vi "Voltage Cycle.vi"() -> ()   [LabVIEW 2015]
uses:
  <instrlib>/Agilent E363X Series/Agilent E363X Series.lvlib
panel:
  in  "Delay Control":dbl format="%#_g seconds"
  in  "Ending Voltage":dbl format="%#_g V"
  in  "Voltage Step":dbl format="%#_g V"
  out "# Trials":dbl
  in  "Dosimeter Id":string
  in  "Starting Voltage":dbl format="%#_g V"
  out "?":bool
  in  "Current Limit (1.0 A)":dbl=1.0 format="%.3g"
  out "Actual Current Level (A)":dbl format="%.3g"
  in  "Channel (1: Channel 1)":i32(ring)=1 items=["Channel 1"=1, "Channel 2"=2, "Channel 3"=3]
  out "Actual Voltage Level (V)":dbl format="%.3g"
  in  "VISA resource name":refnum<visa-resource-name>
  in  "?":bool
  in  "# Measurements":dbl format="%#_g "
  in  "Time inbetween Trials":dbl format="%#_g seconds"
  in  "Time inbetween Measurements":dbl format="%#_g seconds"
  out "Output":string="Start Ipad"
  out "Voltage":dbl(knob) scale=0.0..6.0
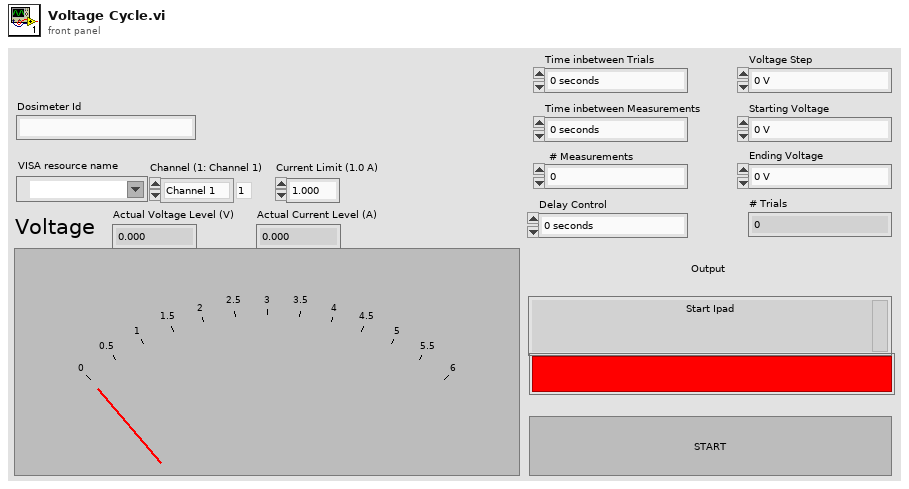
[diagram p1: front panel]
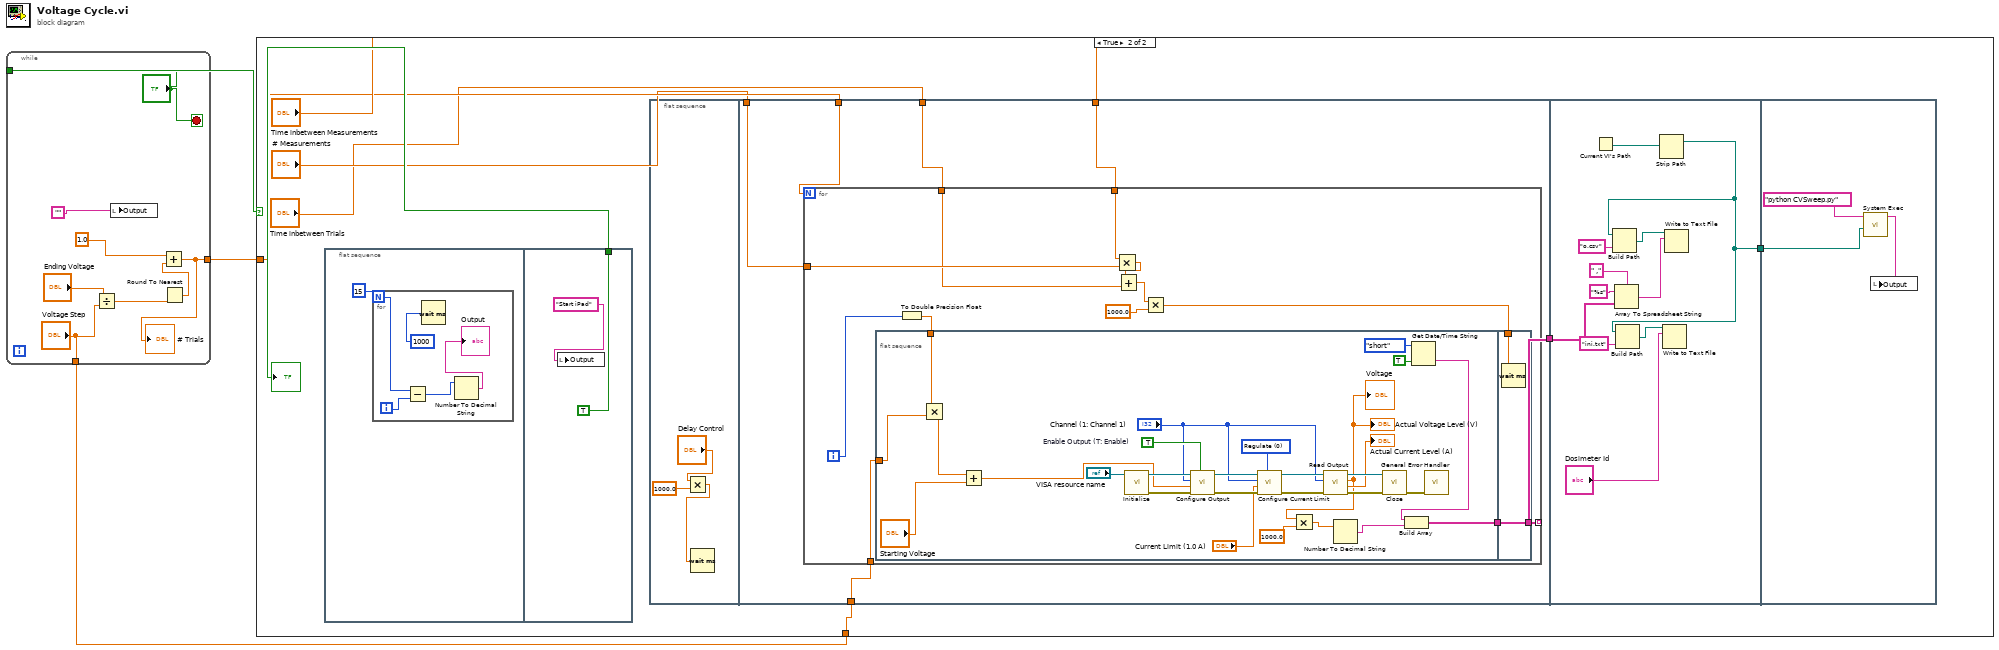
[diagram p0: block diagram]
diagram:
  n1 = while {
    tunnel: ["?"] -> w3
    tunnel: [w5] -> w2
    tunnel: ["Voltage Step"] -> w1
    stop <- "?" stop-if-true
    n2 = Divide(x="Ending Voltage", y="Voltage Step") -> (x/y=w8:dbl)
    n3 = local write "Output"("") -> ()
    n4 = Round To Nearest(number=w8) -> (nearest integer value=w6:dbl)
    n5 = Add(x=1.0, y=w6) -> (x+y=w5:dbl)
    "# Trials" <- w5
  }
  n6 = case shown="True" w3 {
    tunnel: w2 -> [_ w15]
    tunnel: w1 -> [_ w12]
    frame False {
    }
    frame True {
      n7 = flat-sequence {
        tunnel: [TRUE] -> w19
        frame #0 {
          n8 = for {
            N: 15 -> [w90]
            i -> [w89]
            n9 = Subtract(x=w90, y=w89) -> (x-y=w88:i32)
            n10 = Wait (ms)(milliseconds to wait=u32 1000) -> ()  [unwired: 1 out]
            n11 = Number To Decimal String(number=w88) -> (decimal integer string=→"Output":string)  [unwired: 1 in]
          }
        }
        frame #1 {
          n12 = local write "Output"("Start iPad") -> ()
        }
      }
      n13 = flat-sequence {
        tunnel: "Time inbetween Measurements" -> [w28]
        tunnel: [w27] -> w17
        tunnel: w15 -> [w23]
        tunnel: "# Measurements" -> [w26]
        tunnel: "Time inbetween Trials" -> [w25]
        tunnel: w12 -> [w24]
        tunnel: w17 -> [w76]
        tunnel: [w71] -> w16
        tunnel: w16 -> [w83]
        frame #0 {
          n14 = Multiply(x="Delay Control", y=1000.0) -> (x*y=w20:dbl)
          n15 = Wait (ms)(milliseconds to wait=w20) -> ()  [unwired: 1 out]
        }
        frame #1 {
          n16 = for {
            N: w23 -> [_]
            tunnel: [w39] -> w27 mode=indexing
            tunnel: w28 -> [w34]
            tunnel: w26 -> [w33]
            tunnel: w25 -> [w32]
            tunnel: w24 -> [w31]
            i -> [w29]
            n17 = flat-sequence {
              tunnel: [w47] -> w36
              tunnel: w31 -> [w42]
              tunnel: w30 -> [w41]
              tunnel: [w70] -> w39
              tunnel: w36 -> [w70]
              tunnel: w35 -> [w69]
              frame #0 {
                w54 = u16 0 items=["Regulate", "Trip"] ("Behavior (0: Regulate)")
                w64 = TRUE  # Enable Output (T: Enable)
                n18 = Multiply(x=w41, y=w42) -> (x*y=w52:dbl)
                n19 = Add(x=w52, y="Starting Voltage") -> (x+y=w51:dbl)
                n20 = call <instrlib>:"Initialize.vi"("VISA resource name"="VISA resource name") -> ("error out"=w65:errorcluster, "VISA resource name out"=w67:refnum<visa-resource-name>)  [unwired: 9 in]
                n21 = call <instrlib>:"Configure Output.vi"("Enable Output (T: Enable)"=w64, "error in (no error)"=w65, "Voltage Level (0.0 V)"=w51, "Channel (1: Channel 1)"="Channel (1: Channel 1)", "VISA resource name"=w67) -> ("error out"=w59:errorcluster, "VISA resource name out"=w60:refnum<visa-resource-name>)  [unwired: 5 in]
                n22 = call <instrlib>:"Configure Current Limit.vi"("Behavior (0: Regulate)"=w54, "error in (no error)"=w59, "Current Limit (0.0 A)"="Current Limit (1.0 A)", "Channel (1: Channel 1)"="Channel (1: Channel 1)", "VISA resource name"=w60) -> ("error out"=w58:errorcluster, "VISA resource name out"=w57:refnum<visa-resource-name>)  [unwired: 5 in]
                n23 = call <instrlib>:"Read Output.vi"("error in (no error)"=w58, "Channel (1: Channel 1)"="Channel (1: Channel 1)", "VISA resource name"=w57) -> ("error out"=w63:errorcluster, "Actual Current Level (A)"=→"Actual Current Level (A)":dbl, "Actual Voltage Level (V)"=w45:dbl, "VISA resource name out"=w62:refnum<visa-resource-name>)  [unwired: 5 in]
                "Voltage" <- w45
                "Actual Voltage Level (V)" <- w45
                n24 = Multiply(x=w45, y=1000.0) -> (x*y=w43:dbl)
                n25 = Number To Decimal String(number=w43) -> (decimal integer string=w46:string)  [unwired: 1 in]
                n26 = call <instrlib>:"Close.vi"("error in (no error)"=w63, "VISA resource name"=w62) -> ("error out"=w66:errorcluster)  [unwired: 9 in]
                n27 = Get Date/Time String(date format (0)=enum16{"short", "long", "abbreviated"}."short", want seconds? (F)=TRUE) -> (time string=w48:string)  [unwired: 1 in, 1 out]
                n28 = Build Array(w48, w46) -> (w47:string[])
                n29 = call <vilib>:"General Error Handler.vi"("error in (no error)"=w66) -> ()  [unwired: 10 in, 5 out]
              }
              frame #1 {
                n30 = Wait (ms)(milliseconds to wait=w69) -> ()  [unwired: 1 out]
              }
            }
            n31 = To Double Precision Float(number=w29) -> (double precision float=w30:dbl)
            n32 = Multiply(x=w34, y=w33) -> (x*y=w40:dbl)
            n33 = Add(x=w40, y=w32) -> (x+y=w38:dbl)
            n34 = Multiply(x=w38, y=1000.0 ("x")) -> (x*y=w35:dbl)
          }
        }
        frame #2 {
          n35 = Current VI's Path() -> (path=w72:path)
          n36 = Array To Spreadsheet String(delimiter (Tab)=" ,", array=w76, 3:"%s" ("format string")) -> (spreadsheet string=w79:string)
          n37 = Strip Path(path=w72) -> (stripped path=w71:path)  [unwired: 1 out]
          n38 = Build Path(base path=w71, name or relative path="o.csv") -> (appended path=w80:path)
          n39 = Build Path(base path=w71, name or relative path="ini.txt") -> (appended path=w74:path)
          n40 = Write to Text File(file (use dialog)=w74, text="Dosimeter Id") -> ()  [unwired: 2 in, 3 out]
          n41 = Write to Text File(file (use dialog)=w80, text=w79) -> ()  [unwired: 2 in, 3 out]
        }
        frame #3 {
          n42 = call <vilib>:"System Exec.vi"("working directory"=w83, "command line"="python CVSweep.py") -> ("standard output"=w82:string)  [unwired: 6 in, 3 out]
          n43 = local write "Output"(w82) -> ()
        }
      }
      "?" <- w19
    }
  }
